vi "Flywheel_Execute.vi"() -> ()   [LabVIEW 2019]
uses:
  Globals/Flywheel_Globals.vi
  Globals/Sensor_Values.vi
  Utility VIs/Basic_Motor_Modes.ctl
panel:
  in  "array 2":dbl[][](array[numeric])
  in  "array":dbl[][](array[numeric])
  out "added Area":dbl=-0.27951836585998535
  in  "Camera Area D":dbl=17.0
  in  "Default_Flywheel_Speed":dbl=4750.0
  in  "Flywheel_MaxSpeed(RPM)":dbl=4900.0
  out "Camera_Area":dbl=1.2052602767944336
  out "Error":cluster{dbl, dbl}(graph)
  out "Spun-Up":bool
  out "Error":dbl
  in  "Acceptable_error":dbl=200.0
  # "Click here to set min"
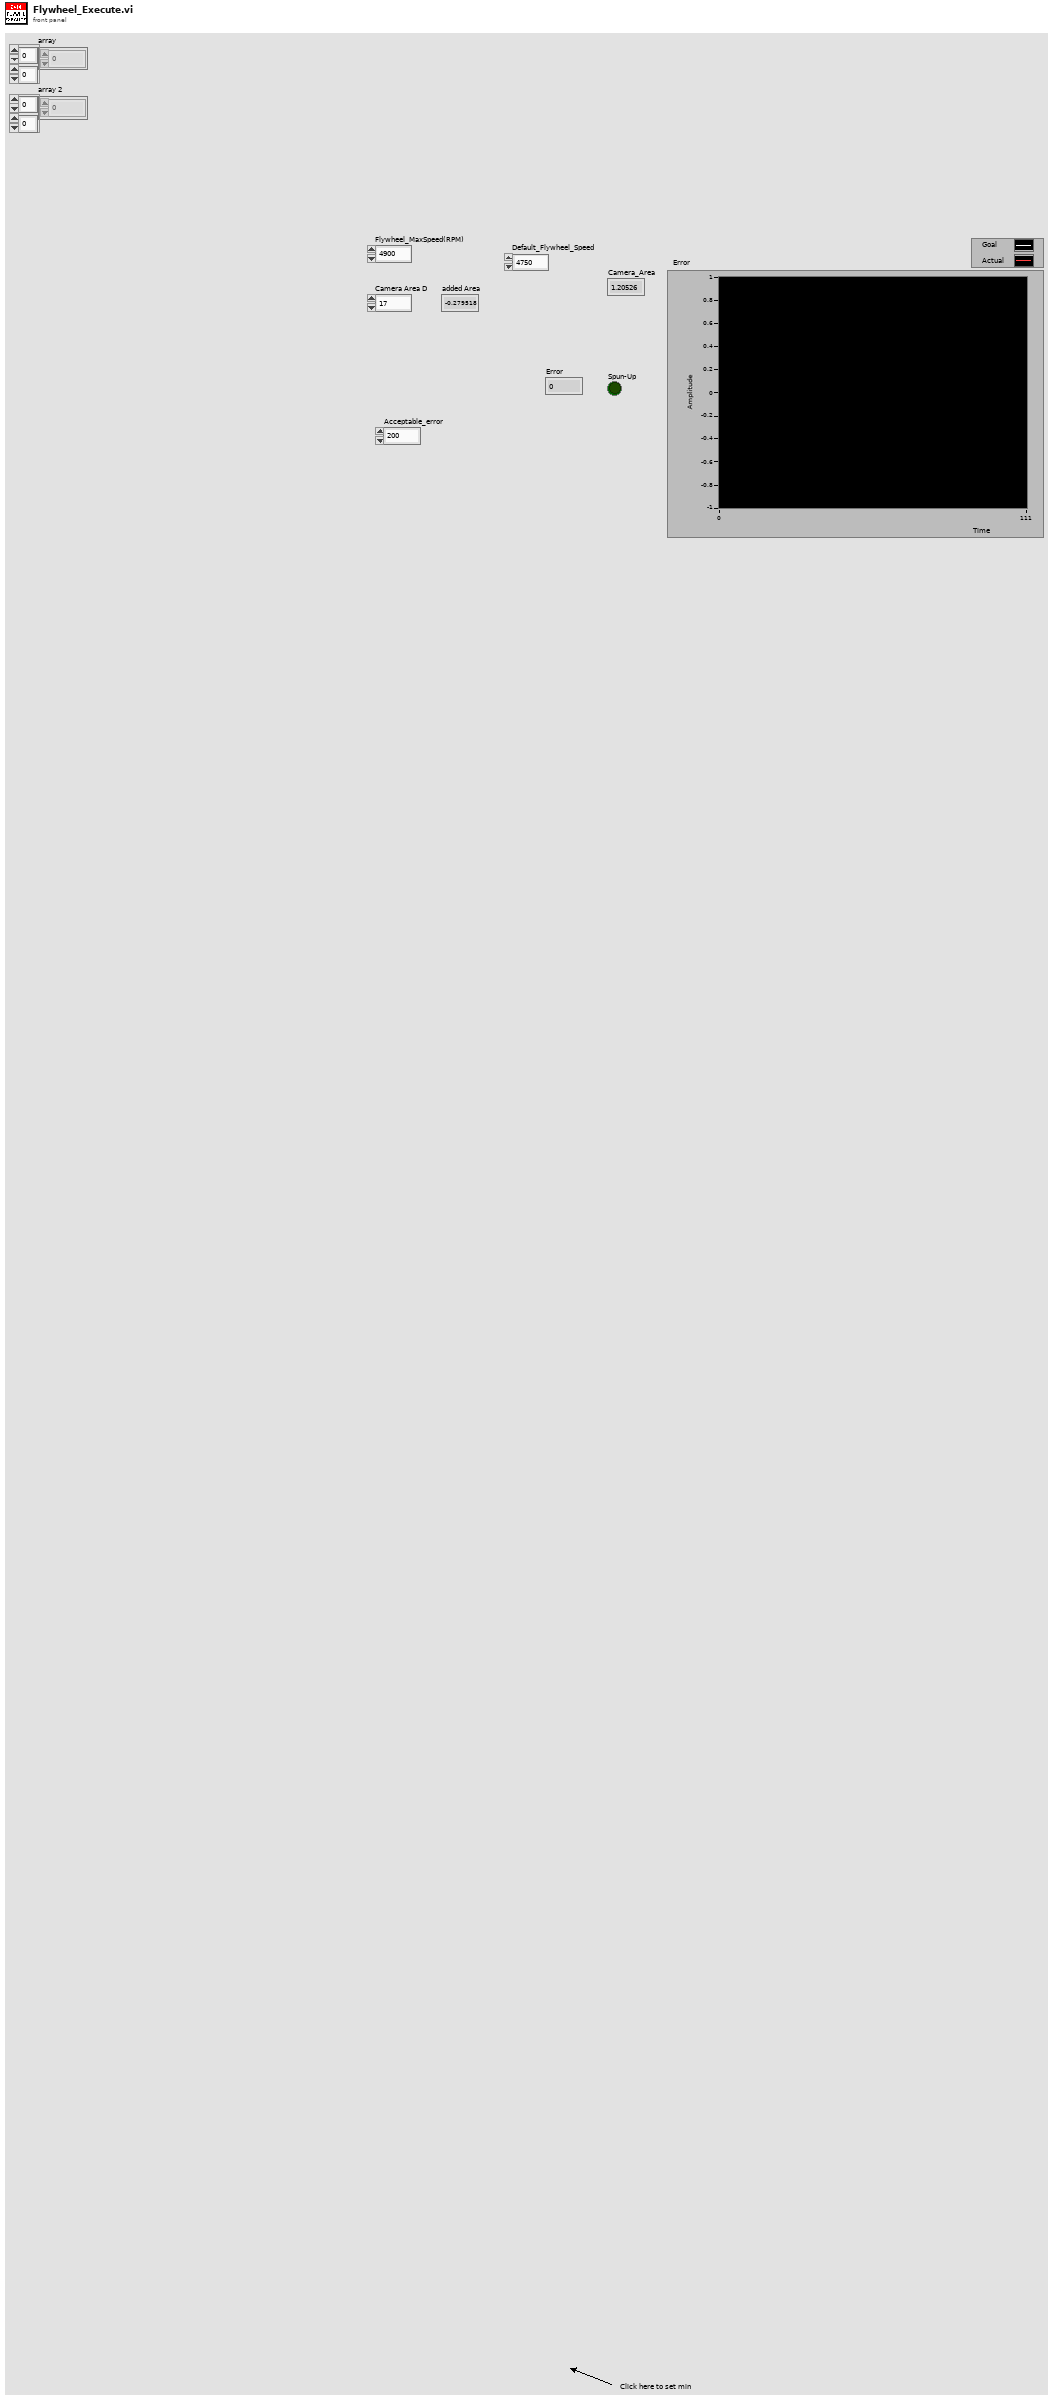
[diagram p1: front panel]
types:
  T1 = typedef "Basic_Motor_Modes.ctl" = enum16{"Percent_Voltage", "Speed_Control", "Position_Control", "Current"}
  T2 = typedef "Flywheel_Cluster.ctl" = cluster{"Flywheel_Throttle":dbl, "Control_States":T3, "Auto_Speed":bool, "Flywheel_On":bool, "Auto_Notifier":refnum<notifier>, "Step":dbl, "Parameters":dbl[]}
  T3 = typedef "Flywheel_States.ctl" = enum16{"No-Op", "Percent_Voltage", "Speed_Control_Manual", "Speed_Control_Auto", "Command_SpinUp", "Command_SpinUpAuto"}
  T4 = cluster{"Flywheel_Output":dbl, "Flywheel_Velocity(RPM)":dbl}
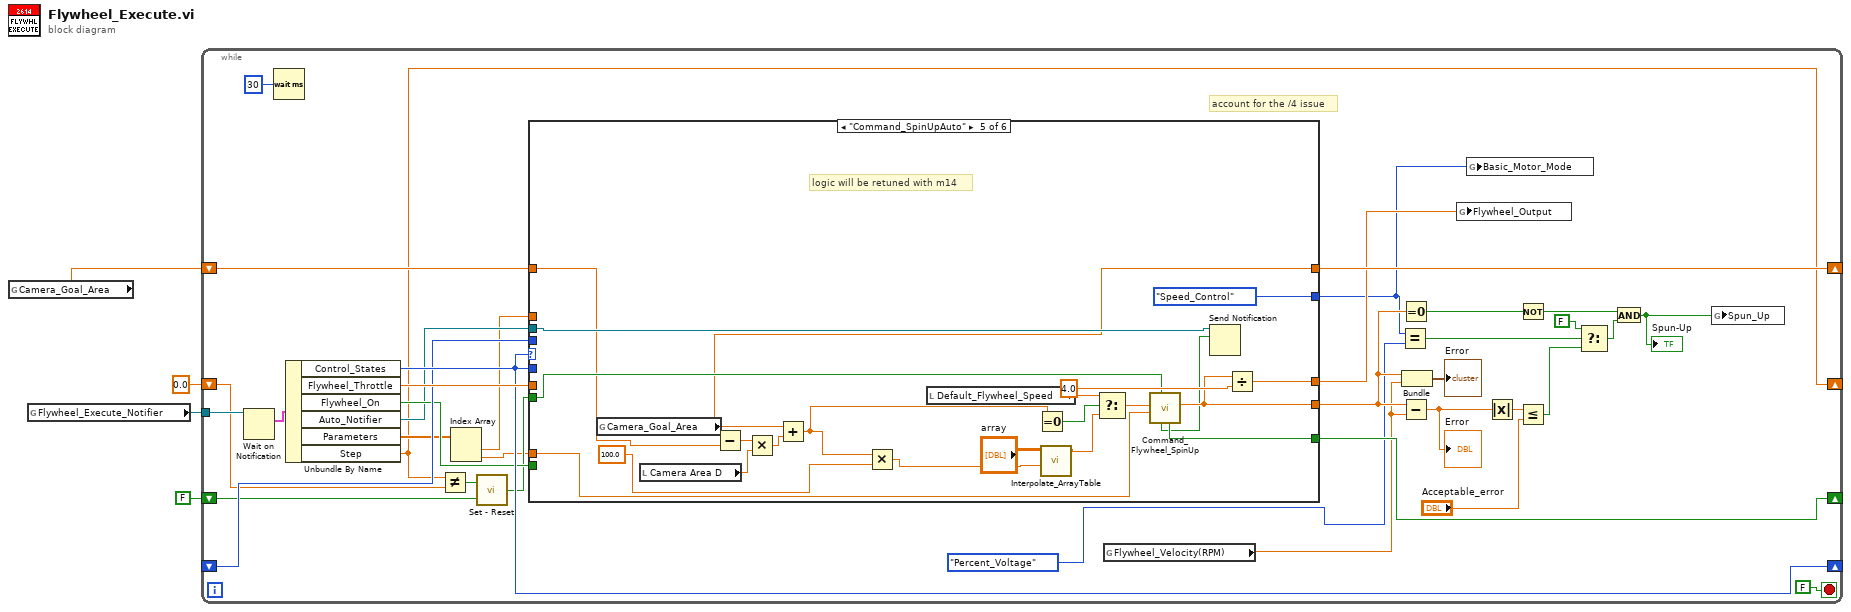
[diagram p0: block diagram]
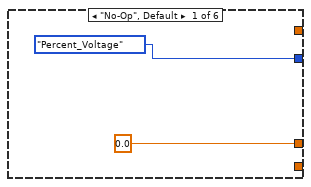
[diagram p2: hidden frame]
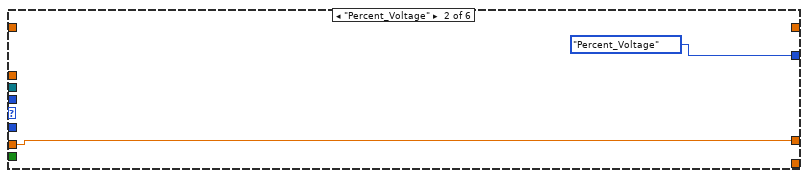
[diagram p3: hidden frame]
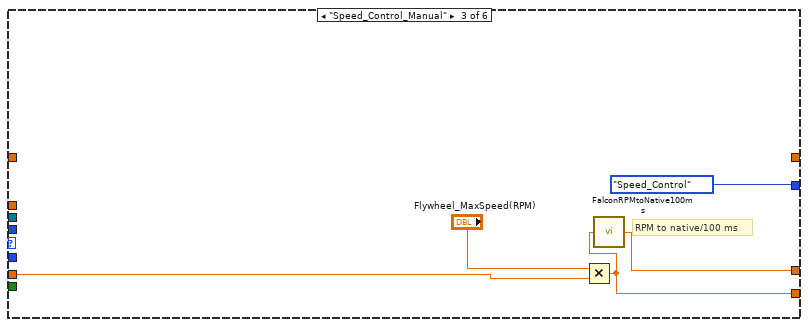
[diagram p4: hidden frame]
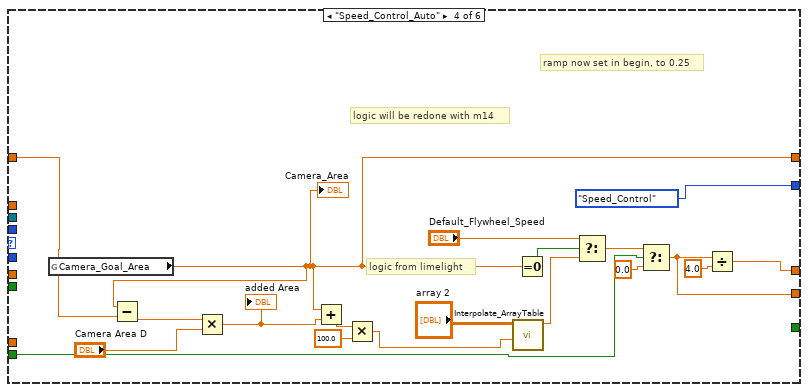
[diagram p5: hidden frame]
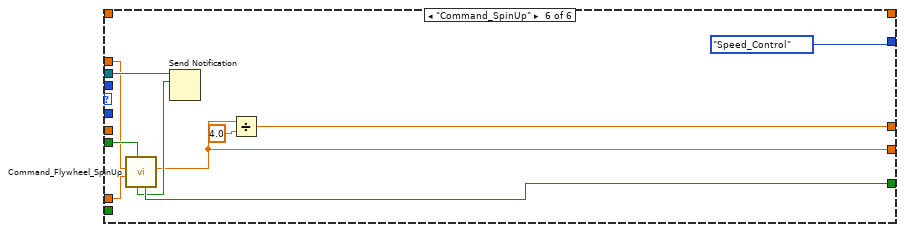
[diagram p6: hidden frame]
diagram:
  n1 = global read "Sensor_Values.vi" "Camera_Goal_Area"() -> (w1:dbl)
  n2 = global read "Flywheel_Globals.vi" "Flywheel_Execute_Notifier"() -> (w4:refnum<notifier>)
  n3 = while {
    tunnel: w4 -> [w39]
    shift-right: [w35] -> _
    shift-left: _ -> [w34]
    shift-right: [w5] -> _
    shift-left: 0.0 ("Step") -> [w14]
    shift-right: [w18] -> _
    shift-left: FALSE ("Reint") -> [w19]
    shift-right: [w12] -> _
    shift-left: w1 -> [w13]
    stop <- FALSE stop-if-true
    # "account for the /4 issue"
    n4 = Wait on Notification(notifier=w39) -> (notification=w38:T2)  [unwired: 3 in, 3 out]
    n5 = Wait (ms)(milliseconds to wait=u32 30) -> ()  [unwired: 1 out]
    n6 = Unbundle By Name(w38) -> ("Control_States"=w35:T3, "Flywheel_Throttle"=w37:dbl, "Flywheel_On"=w23:bool, "Auto_Notifier"=w17:refnum<notifier>, "Parameters"=w16:dbl[], "Step"=w5:dbl)
    n7 = Not Equal?(x=w5, y=w14) -> (x != y?=w15:bool)
    n8 = Index Array(array=w16) -> (element #1=w7:dbl, element #2=w6:dbl)  [unwired: 2 in]
    n9 = call "Set - Reset.vi"("Reset"=w19, "Set"=w15) -> ("Output"=w20:bool)
    n10 = case shown="\"Command_SpinUpAuto\"" w35 {
      tunnel: [0.0 ("Flywheel_Throttle") w44 w45 w68 w89 w94] -> w11
      tunnel: w37 -> [_ w44 w49 _ _ _]
      tunnel: w35 -> [_ _ _ _ _ _]
      tunnel: w34 -> [_ _ _ _ _ _]
      tunnel: [_ _ w46 w67 w84 w92] -> w25
      tunnel: w23 -> [_ _ _ w66 _ _]
      tunnel: w20 -> [_ _ _ _ w82 w100]
      tunnel: [_ _ _ _ w81 w99] -> w18
      tunnel: w17 -> [_ _ _ _ w80 w98]
      tunnel: w7 -> [_ _ _ _ _ w96]
      tunnel: w6 -> [_ _ _ _ w83 w95]
      tunnel: w13 -> [_ _ _ w58 w71 _]
      tunnel: [_ _ _ w53 w75 _] -> w12
      tunnel: [Basic_Motor_Modes."Percent_Voltage" ("Motor_Mode") Basic_Motor_Modes."Percent_Voltage" ("Motor_Mode") Basic_Motor_Modes."Speed_Control" ("Motor_Mode") Basic_Motor_Modes."Speed_Control" ("Motor_Mode") Basic_Motor_Modes."Speed_Control" ("Motor_Mode") Basic_Motor_Modes."Speed_Control" ("Motor_Mode")] -> w9
      frame "No-Op", Default {
      }
      frame "Percent_Voltage" {
      }
      frame "Speed_Control_Manual" {
        # "RPM to native/100 ms"
        n11 = Multiply(x="Flywheel_MaxSpeed(RPM)", y=w49) -> (x*y=w46:dbl)
        n12 = call "FalconRPMtoNative100ms.vi"("RPM"=w46) -> ("raw sensor units / 100 ms"=w45:dbl)  [unwired: 4 in]
      }
      frame "Speed_Control_Auto" {
        # "logic will be redone with m14"
        # "ramp now set in begin, to 0.25"
        # "logic from limelight"
        n13 = global read "Sensor_Values.vi" "Camera_Goal_Area"() -> (w53:dbl)
        "Camera_Area" <- w53
        n14 = Subtract(x=w53, y=w58) -> (x-y=w57:dbl)
        n15 = Multiply(x=w57, y="Camera Area D") -> (x*y=w52:dbl)
        "added Area" <- w52
        n16 = Add(x=w53, y=w52) -> (x+y=w54:dbl)
        n17 = Multiply(x=w54, y=100.0) -> (x*y=w59:dbl)
        n18 = call "Interpolate_ArrayTable.vi"("Desired_Distance"=w59, "array"="array 2") -> ("RPM"=w60:dbl)  [unwired: 9 in]
        n19 = Equal To 0?(x=w53) -> (x = 0?=w63:bool)
        n20 = Select(t="Default_Flywheel_Speed", s=w63, f=w60) -> (s? t:f=w61:dbl)
        n21 = Select(t=w61, s=w66, f=0.0) -> (s? t:f=w67:dbl)
        n22 = Divide(x=w67, y=4.0) -> (x/y=w68:dbl)
      }
      frame "Command_SpinUpAuto" {
        # "logic will be retuned with m14"
        n23 = global read "Sensor_Values.vi" "Camera_Goal_Area"() -> (w75:dbl)
        n24 = local read "Camera Area D"() -> (w72:dbl)
        n25 = Subtract(x=w75, y=w71) -> (x-y=w74:dbl)
        n26 = Multiply(x=w74, y=w72) -> (x*y=w73:dbl)
        n27 = Add(x=w75, y=w73) -> (x+y=w76:dbl)
        n28 = Multiply(x=w76, y=100.0) -> (x*y=w77:dbl)
        n29 = local read "Default_Flywheel_Speed"() -> (w86:dbl)
        n30 = Equal To 0?(x=w76) -> (x = 0?=w87:bool)
        n31 = call "Interpolate_ArrayTable.vi"("Desired_Distance"=w77, "array"="array") -> ("RPM"=w78:dbl)  [unwired: 9 in]
        n32 = Select(t=w86, s=w87, f=w78) -> (s? t:f=w85:dbl)
        n33 = call "Command_Flywheel_SpinUp.vi"("Startup"=w82, "Timeout"=w83, "Speed"=w85) -> ("Flywheel_Output"=w84:dbl, "Reint"=w81:bool, "Completed"=w79:bool)  [unwired: 6 in]
        n34 = Send Notification(notification=w79, notifier=w80) -> ()  [unwired: 1 in, 2 out]
        n35 = Divide(x=w84, y=4.0) -> (x/y=w89:dbl)
      }
      frame "Command_SpinUp" {
        n36 = call "Command_Flywheel_SpinUp.vi"("Startup"=w100, "Timeout"=w95, "Speed"=w96) -> ("Flywheel_Output"=w92:dbl, "Reint"=w99:bool, "Completed"=w97:bool)  [unwired: 6 in]
        n37 = Send Notification(notification=w97, notifier=w98) -> ()  [unwired: 1 in, 2 out]
        n38 = Divide(x=w92, y=4.0) -> (x/y=w94:dbl)
      }
    }
    n39 = global read "Sensor_Values.vi" "Flywheel_Velocity(RPM)"() -> (w8:dbl)
    n40 = Equal?(x=w9, y=Basic_Motor_Modes."Percent_Voltage" ("Motor_Mode")) -> (x = y?=w31:bool)
    n41 = Equal To 0?(x=w25) -> (x = 0?=w28:bool)
    n42 = Subtract(x=w25, y=w8) -> (x-y=w26:dbl)
    "Error" <- w26
    n43 = Bundle("Flywheel_Output"=w25, "Flywheel_Velocity(RPM)"=w8) -> (→"Error":T4)  [unwired: 1 in]
    n44 = global write "Flywheel_Globals.vi" "Flywheel_Output"(w11) -> ()
    n45 = global write "Flywheel_Globals.vi" "Basic_Motor_Mode"(w9) -> ()
    n46 = Absolute Value(x=w26) -> (abs(x)=w33:dbl)
    n47 = Not(x=w28) -> (.not. x?=w27:bool)
    n48 = Less Or Equal?(x=w33, y="Acceptable_error") -> (x <= y?=w29:bool)
    n49 = Select(t=FALSE, s=w31, f=w29) -> (s? t:f=w22:bool)
    n50 = And(x=w27, y=w22) -> (x .and. y?=w21:bool)
    "Spun-Up" <- w21
    n51 = global write "Flywheel_Globals.vi" "Spun_Up"(w21) -> ()
  }
